vi "Create.vi"(8 "error in (no error)":errorcluster) -> (0 "error out":errorcluster, 3 "Plugin Loader out":refnum<class "Plugin Loader.lvclass">)   [LabVIEW 2020]
uses:
  Plugin Loader.lvclass
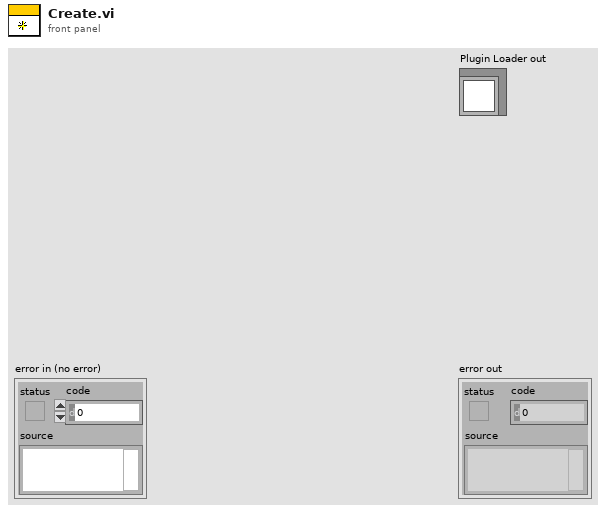
[diagram p1: front panel]
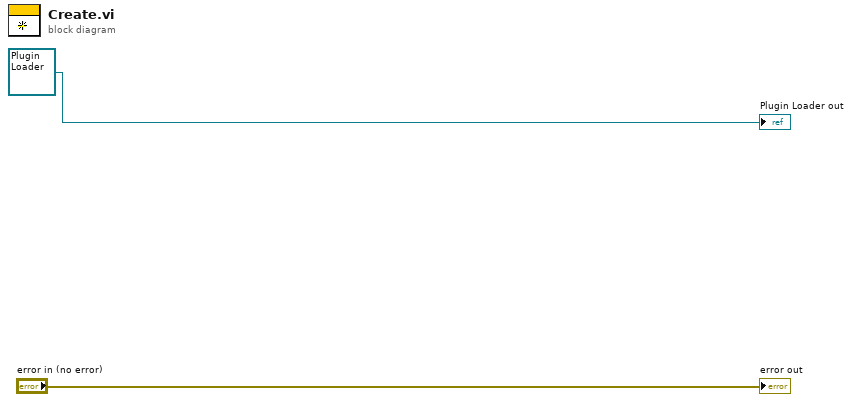
[diagram p0: block diagram]
diagram:
  "error out" <- "error in (no error)"
  "Plugin Loader out" <- refnum<class "Plugin Loader.lvclass"> refnum ("Plugin Loader in")
